vi "Postion Top Bar Units.vi"(7 "Units":refnum<vi>, 8 "Button Size:Height":u32, 9 "Button Witdh":dbl, 10 "Top (numeric indicator)":u32, 11 "Left (numeric indicator)":u32) -> (0 "error out":errorcluster)   [LabVIEW 2014]
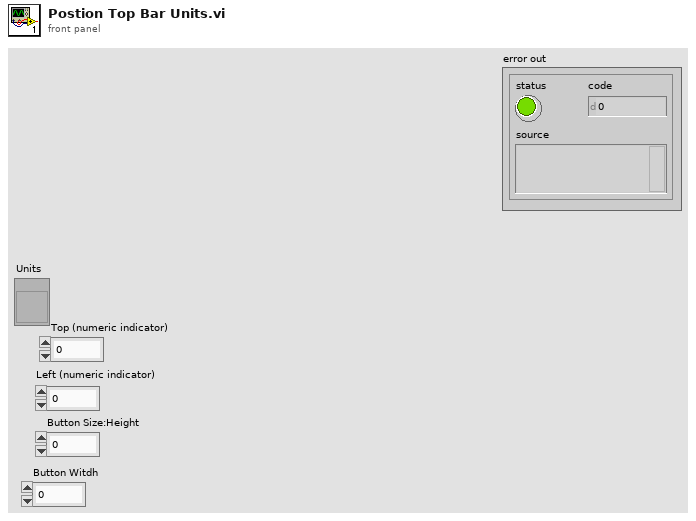
[diagram p1: front panel]
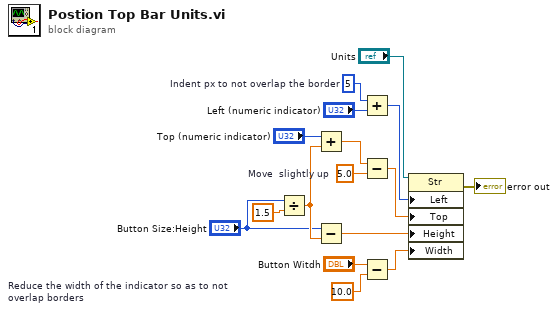
[diagram p0: block diagram]
diagram:
  w1 = 5.0  # Move  slightly up
  w8 = u32 5  # Indent px to not overlap the border
  w10 = 10.0  # Reduce the width of the indicator so as to not overlap borders
  n1 = Divide(x="Button Size:Height", y=1.5) -> (x/y=w13:dbl)
  n2 = Add(x="Top (numeric indicator)", y=w13) -> (x+y=w14:dbl)
  n3 = Subtract(x="Button Size:Height", y=w13) -> (x-y=w12:dbl)
  n4 = Add(x=w8, y="Left (numeric indicator)") -> (x+y=w9:u32)
  n5 = Subtract(x=w14, y=w1) -> (x-y=w2:dbl)
  n6 = Subtract(x="Button Witdh", y=w10) -> (x-y=w11:dbl)
  n7 = property class="Str"(reference="Units", "Left"=w9, "Top"=w2, "Height"=w12, "Width"=w11) -> (error out=→"error out":errorcluster)  [unwired: 1 in, 1 out]
